vi "Initial Program.vi"() -> (3 "Initial Program":T1={"Raw Logging Configuration"={"Log File Base Path"=path "", "Enable Log File"=FALSE}, "Sequence"={"Start RPM"=10.0, "End RPM"=150.0, "# RPM Steps"=10, "Dwell (s)"=10.0, "Start L-value / Resist"=1, "End L-value/Resist"=10, "# L-value/Resist Steps"=10, "Steady State +/-RPM"=10.0, "Enable Steady State +/- RPM"=FALSE, "Steady State Window (s)"=10.0, "Enable Steady State Max Wait"=FALSE, "Max Settle Time (s)"=10.0, "Enable Temperature Rest"=FALSE, "Rest TC2 threshold (degF)"=2.0, "Enable Max Time Rest"=FALSE, "Max Rest Time (s)"=10.0, "Rest RPM"=2.0, "RPM Ramp (rpm/s)"=10.0, "Resistance Motor Mode"=enum."v1 Bike"}, "Summary  CSV Log Configuration"={"Report  CSV File Path"=path "C:/Users/nlim/Documents/LabVIEW Data/Logged Data.tdms", "Enable Report CSV File"=FALSE}, "CSV Log Info"={"Report Title"="", "Time Stamp"=timestamp(0 s since 1904-01-01), "Serial Number"="", "Initial Temperature"=0.0, "Comments"=""}, "Table"=[]} {"Sequence"."RPM Ramp (rpm/s)" min=0.0 format="%#_6f"; "Sequence"."Rest RPM" min=0.0 format="%.1f"; "Sequence"."Max Rest Time (s)" min=0.0 format="%.1f"; "Sequence"."Rest TC2 threshold (degF)" format="%.1f"; "Sequence"."Max Settle Time (s)" min=0.0 format="%.1f"; "Sequence"."Steady State Window (s)" min=0.0 format="%.1f"; "Sequence"."Steady State +/-RPM" min=0.0 format="%.1f"; "Sequence"."# L-value/Resist Steps" min=1; "Sequence"."End L-value/Resist" min=0 max=100; "Sequence"."Start L-value / Resist" min=0 max=100; "Sequence"."Dwell (s)" min=0.0 format="%#_6f"; "Sequence"."# RPM Steps" min=1; "Sequence"."End RPM" min=0.0 max=200.0 format="%#_6f"; "Sequence"."Start RPM" min=0.0 max=200.0 format="%#_6f"})   [LabVIEW 2015, in "Config Module.lvlib"]
uses:
  Config Module.lvlib
  Settings/Program Cluster.ctl
  Logging/Logging Configuration.ctl
  Settings/Sequence Cluster.ctl
  Resistance Motor/Resistance Mode Enum.ctl
  controls/CSV Log Cluster.ctl
  controls/CSV Log Info Cluster.ctl
  <vilib>/Utility/sysdir.llb/System Directory Type.ctl
  Logging/Logging.lvlib
  Settings/Settings.lvlib
panel:
  # "Settled when"
  # "RPM is within"
  # "RPM of set RPM for last"
  # "seconds"
  # "OR"
  # "seconds since last step change"
  # "More than"
  # "Rest at end of each step at"
  # "RPM until"
  # "TC2 temperature is below"
  # "deg F"
  # "OR"
  # "seconds have elapsed"
  # "More than"
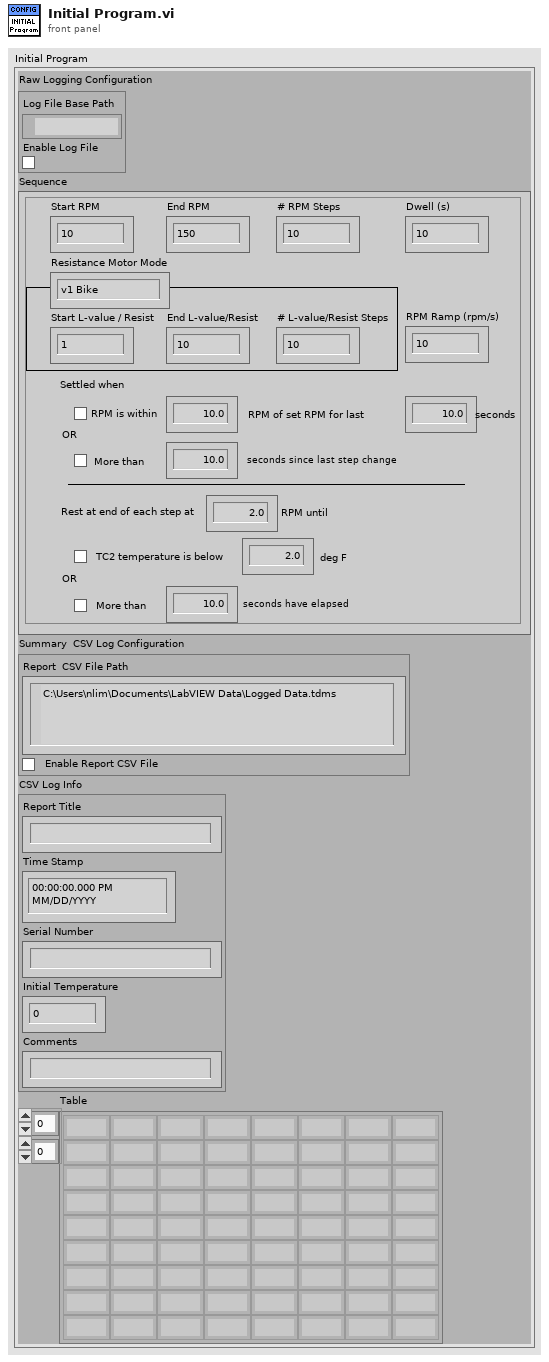
[diagram p1: front panel]
types:
  T1 = typedef "Settings.lvlib/Program Cluster.ctl" = cluster{"Raw Logging Configuration":T2, "Sequence":T3, "Summary  CSV Log Configuration":T5, "CSV Log Info":T6, "Table":string[][]}
  T2 = typedef "Logging.lvlib/Logging Configuration.ctl" = cluster{"Log File Base Path":path, "Enable Log File":bool}
  T3 = typedef "Sequence Cluster.ctl" = cluster{"Start RPM":dbl, "End RPM":dbl, "# RPM Steps":i32, "Dwell (s)":dbl, "Start L-value / Resist":i32, "End L-value/Resist":i32, "# L-value/Resist Steps":i32, "Steady State +/-RPM":dbl, "Enable Steady State +/- RPM":bool, "Steady State Window (s)":dbl, "Enable Steady State Max Wait":bool, "Max Settle Time (s)":dbl, "Enable Temperature Rest":bool, "Rest TC2 threshold (degF)":dbl, "Enable Max Time Rest":bool, "Max Rest Time (s)":dbl, "Rest RPM":dbl, "RPM Ramp (rpm/s)":dbl, "Resistance Motor Mode":T4}
  T4 = typedef "Resistance Mode Enum.ctl" = enum16{"v1 Bike", "v1.5 Bike", "Disabled"}
  T5 = typedef "CSV Log Cluster.ctl" = cluster{"Report  CSV File Path":path, "Enable Report CSV File":bool}
  T6 = typedef "CSV Log Info Cluster.ctl" = cluster{"Report Title":string, "Time Stamp":timestamp, "Serial Number":string, "Initial Temperature":dbl, "Comments":string}
  T7 = typedef "System Directory Type.ctl" = i32
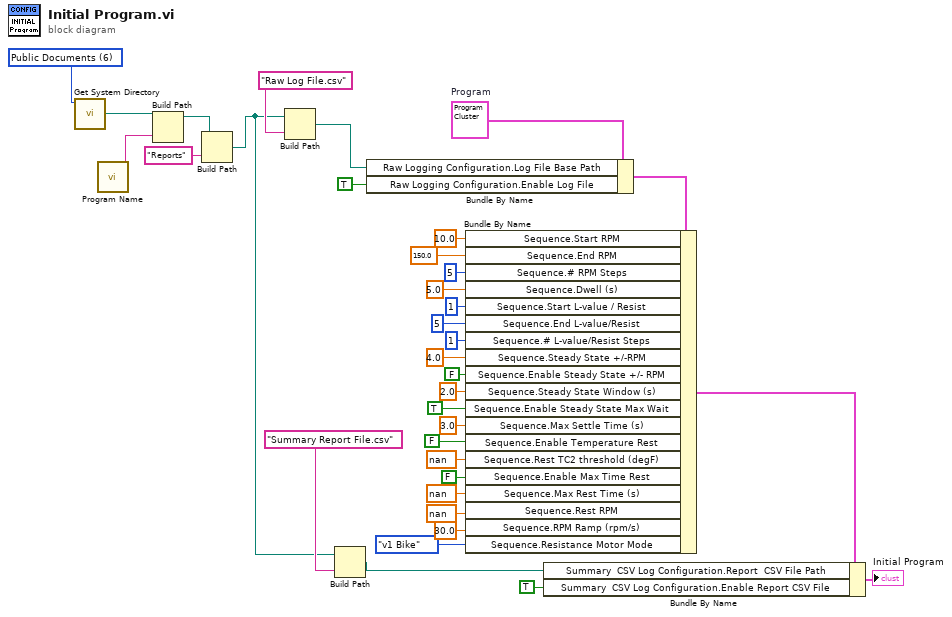
[diagram p0: block diagram]
diagram:
  w19 = T7 6 items=["User Home"=0, "User Desktop"=1, "User Documents"=2, "User Application Data"=3, "User Preferences"=4, "User Temporary"=5, "Public Documents"=6, "Public Application Data"=7, "Public Preferences"=8, "Public Cache"=13, "System Core Libraries"=9, "System Installed Libraries"=10, "Application Files"=11, "Boot Volume Root"=12] ("system directory type")
  w35 = T1 {"Raw Logging Configuration"={"Log File Base Path"=path "", "Enable Log File"=FALSE}, "Sequence"={"Start RPM"=10.0, "End RPM"=150.0, "# RPM Steps"=1, "Dwell (s)"=2.0, "Start L-value / Resist"=0, "End L-value/Resist"=0, "# L-value/Resist Steps"=0, "Steady State +/-RPM"=10.0, "Enable Steady State +/- RPM"=FALSE, "Steady State Window (s)"=10.0, "Enable Steady State Max Wait"=FALSE, "Max Settle Time (s)"=10.0, "Enable Temperature Rest"=FALSE, "Rest TC2 threshold (degF)"=2.0, "Enable Max Time Rest"=FALSE, "Max Rest Time (s)"=10.0, "Rest RPM"=2.0, "RPM Ramp (rpm/s)"=10.0, "Resistance Motor Mode"=enum."v1 Bike"}, "Summary  CSV Log Configuration"={"Report  CSV File Path"=path "C:/Users/nlim/Documents/LabVIEW Data/Logged Data.tdms", "Enable Report CSV File"=FALSE}, "CSV Log Info"={"Report Title"="", "Time Stamp"=timestamp(0 s since 1904-01-01), "Serial Number"="", "Initial Temperature"=0.0, "Comments"=""}, "Table"=[]}  # Program
  n1 = call <vilib>:"Get System Directory.vi"("system directory type"=w19) -> ("system directory"=w18:path)  [unwired: 10 in]
  n2 = call "Program Name.vi"() -> ("Program Name"=w17:string)  [unwired: 11 in]
  n3 = Build Path(base path=w18, name or relative path=w17) -> (appended path=w2:path)
  n4 = Build Path(base path=w2, name or relative path="Reports") -> (appended path=w1:path)
  n5 = Build Path(base path=w1, name or relative path="Raw Log File.csv" ("format string")) -> (appended path=w15:path)
  n6 = Build Path(base path=w1, name or relative path="Summary Report File.csv" ("format string")) -> (appended path=w12:path)
  n7 = Bundle By Name(cluster=w35, "Raw Logging Configuration.Log File Base Path"=w15, "Raw Logging Configuration.Enable Log File"=TRUE ("Logging Configuration.Enable Log File")) -> (w34:T1)
  n8 = Bundle By Name(cluster=w34, "Sequence.Start RPM"=10.0, "Sequence.End RPM"=150.0, "Sequence.# RPM Steps"=5, "Sequence.Dwell (s)"=5.0, "Sequence.Start L-value / Resist"=1 ("Sequence.Start L-value"), "Sequence.End L-value/Resist"=5 ("Sequence.End L-value"), "Sequence.# L-value/Resist Steps"=1 ("Sequence.# L-value Steps"), "Sequence.Steady State +/-RPM"=4.0, "Sequence.Enable Steady State +/- RPM"=FALSE, "Sequence.Steady State Window (s)"=2.0, "Sequence.Enable Steady State Max Wait"=TRUE, "Sequence.Max Settle Time (s)"=3.0 ("Sequence.Steady State Max Wait (s)"), "Sequence.Enable Temperature Rest"=FALSE, "Sequence.Rest TC2 threshold (degF)"=nan, "Sequence.Enable Max Time Rest"=FALSE, "Sequence.Max Rest Time (s)"=nan, "Sequence.Rest RPM"=nan, "Sequence.RPM Ramp (rpm/s)"=30.0 ("Sequence.RPM Ramp (rpm/s/s)"), "Sequence.Resistance Motor Mode"=Resistance_Mode_Enum."v1 Bike") -> (w33:T1)
  n9 = Bundle By Name(cluster=w33, "Summary  CSV Log Configuration.Report  CSV File Path"=w12, "Summary  CSV Log Configuration.Enable Report CSV File"=TRUE) -> (→"Initial Program":T1)
